vi "IsStarboard.vi"(8 "error in (no error)":errorcluster, 10 "Boat Heading (Deg.)":dbl, 11 "Angle in":refnum<class "Angle.lvclass">) -> (0 "error out":errorcluster, 2 "IsStarboard":bool)   [LabVIEW 2013]
doc: "Take in angle, robot heading, returns a boolean \"Is Starboard\", 0 or 1"
uses:
  Angle.lvclass
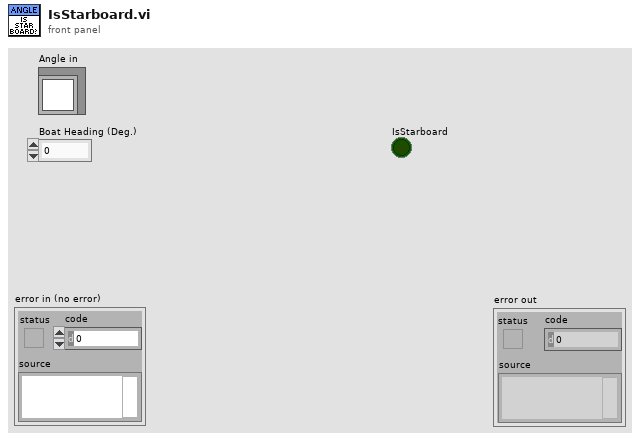
[diagram p1: front panel]
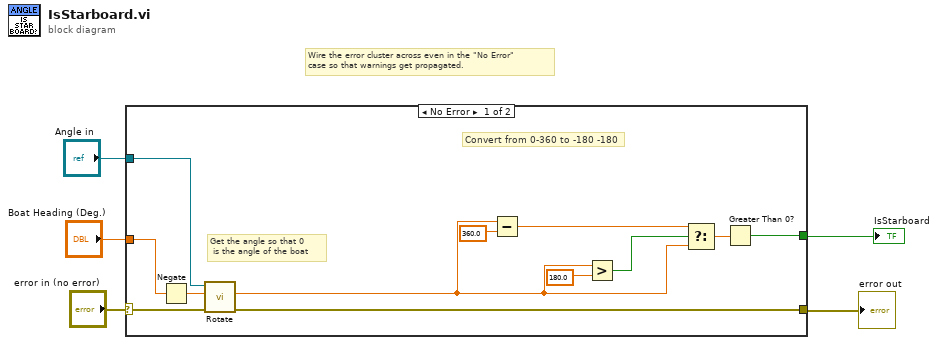
[diagram p0: block diagram]
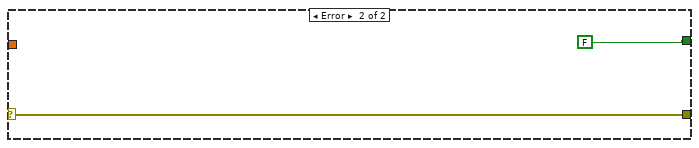
[diagram p2: hidden frame]
diagram:
  # "Wire the error cluster across even in the \"No Error\"\ncase so that warnings get propagated."
  n1 = case shown="No Error" "error in (no error)" {
    selector: "error in (no error)" -> [w17 w19]
    tunnel: [w16 w19] -> w4
    tunnel: "Angle in" -> [w15 _]
    tunnel: [w6 FALSE] -> w2
    tunnel: "Boat Heading (Deg.)" -> [w8 _]
    frame No Error {
      # "Convert from 0-360 to -180 -180"
      # "Get the angle so that 0\n is the angle of the boat"
      n2 = Negate(x=w8) -> (-x=w9:dbl)
      n3 = call "Rotate.vi"("error in (no error)"=w17, "Rotation Angle (Deg.)"=w9, "Angle in"=w15) -> ("error out"=w16:errorcluster, "New Angle"=w10:dbl)  [unwired: 6 in, 1 out]
      n4 = Subtract(x=w10, y=360.0) -> (x-y=w12:dbl)
      n5 = Greater?(x=w10, y=180.0) -> (0:w14:bool)
      n6 = Select(t=w12, s=w14, f=w10) -> (s? t:f=w7:dbl)
      n7 = Greater Than 0?(x=w7) -> (x > 0?=w6:bool)
    }
    frame Error {
    }
  }
  "error out" <- w4
  "IsStarboard" <- w2
